vi "Cast Sensor Data.vi"(5 "SubPort":i32, 6 "Signal Type":enum16{"Digital", "Analog"}(ring), 7 "Port":i32, 8 "error IN":errorcluster, 9 "Key":string, 10 "Modbus Reading":u16[](array[numeric]), 11 "Data IN":map{string, dbl}(c390)) -> (0 "error OUT":errorcluster, 3 "Data OUT":map{string, dbl}(c390))   [LabVIEW 2024, in "IOLink.lvlib"]
uses:
  IOLink.lvlib
panel:
  out "Invalid":bool
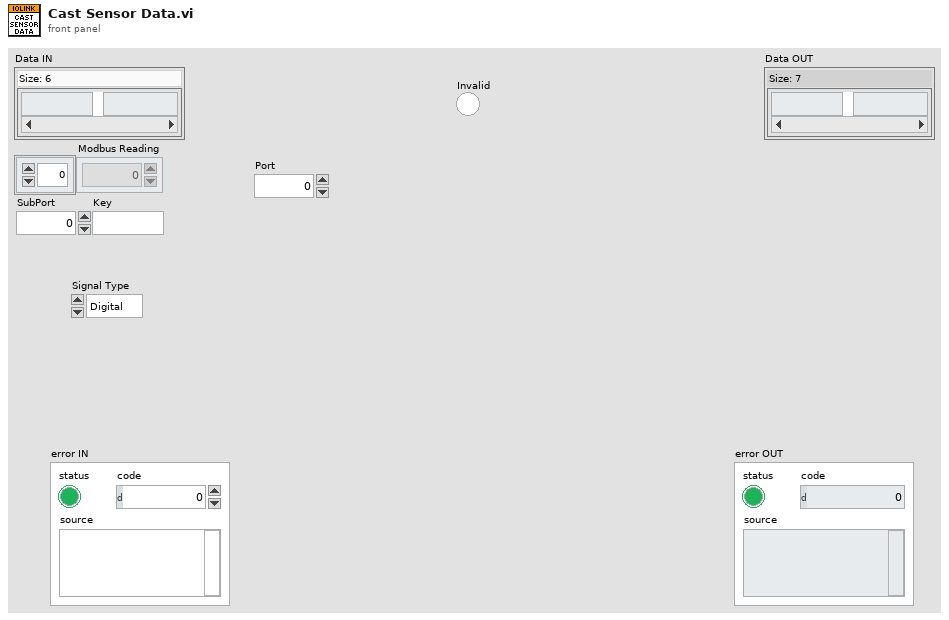
[diagram p1: front panel]
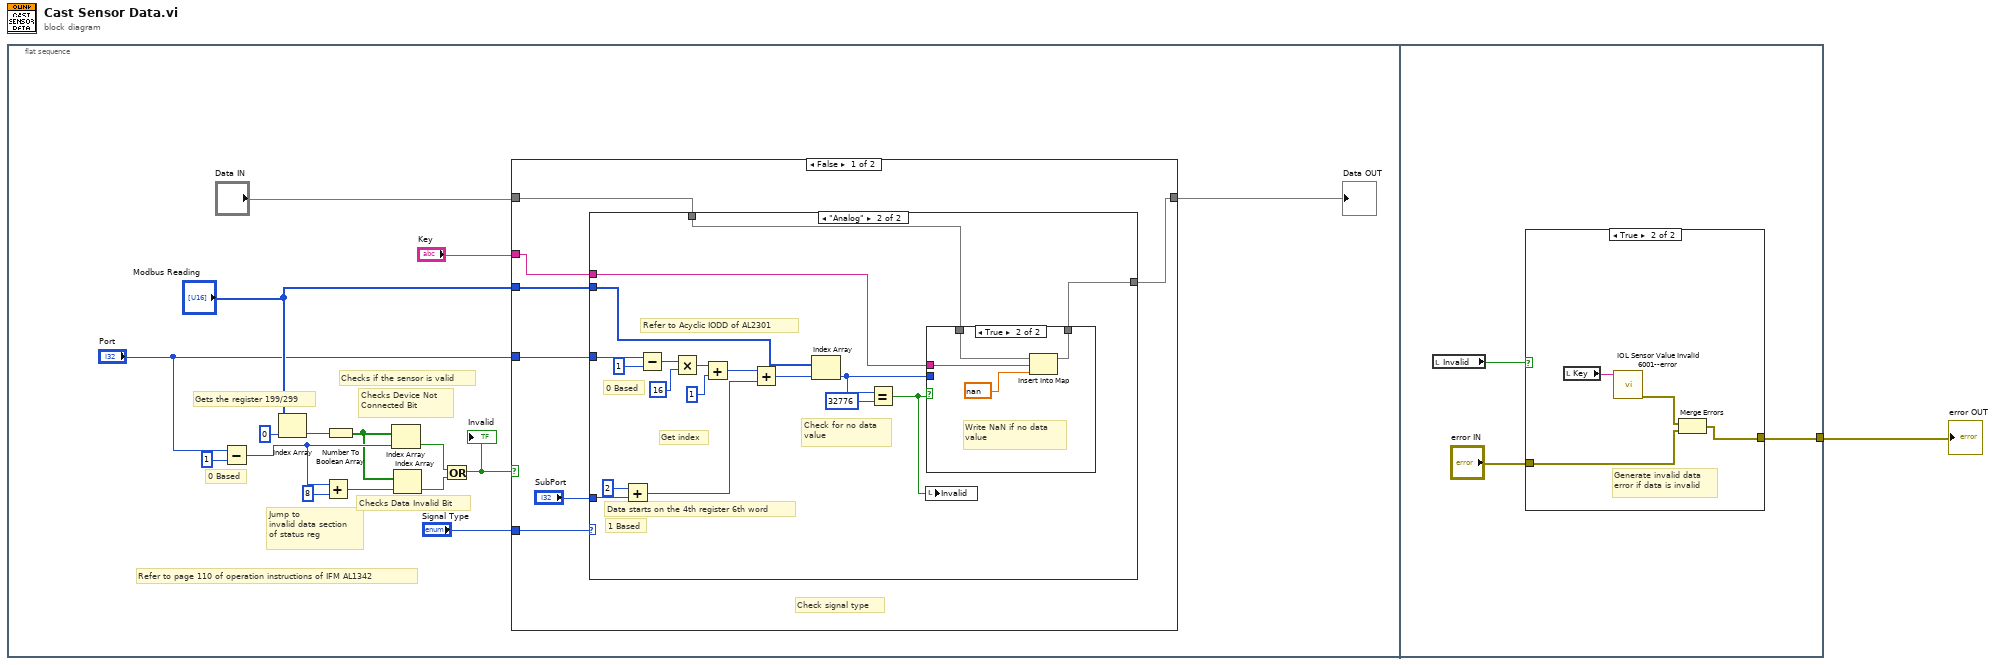
[diagram p0: block diagram]
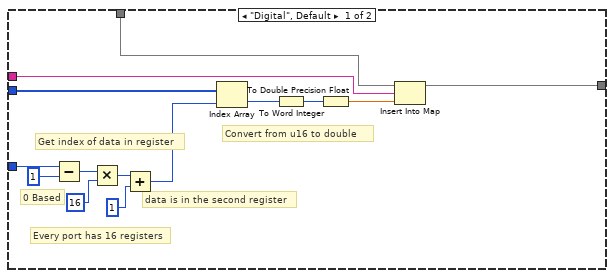
[diagram p2: hidden frame]
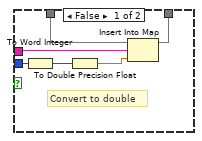
[diagram p3: hidden frame]
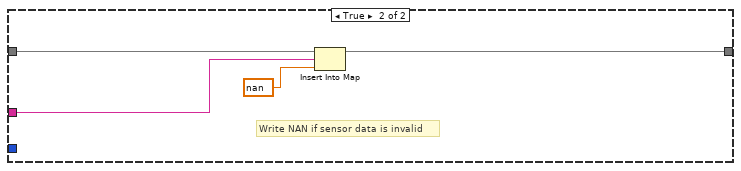
[diagram p4: hidden frame]
diagram:
  n1 = flat-sequence {
    tunnel: [w71] -> w1
    frame #0 {
      # "Checks Data Invalid Bit"
      # "Checks Device Not\nConnected Bit"
      # "Refer to page 110 of operation instructions of IFM AL1342"
      # "Jump to \ninvalid data section\nof status reg"
      # "0 Based"
      # "Gets the register 199/299"
      # "Checks if the sensor is valid"
      n2 = Subtract(x="Port", y=1) -> (x-y=w14:i32)
      n3 = Index Array(array="Modbus Reading", index=0) -> (element=w12:u16)
      n4 = Add(x=w14, y=8) -> (x+y=w15:i32)
      n5 = Number To Boolean Array(number=w12) -> (Boolean array=w13:bool[])
      n6 = Index Array(array=w13, index=w14) -> (element=w16:bool)
      n7 = Index Array(array=w13, index=w15) -> (element=w17:bool)
      n8 = Or(x=w16, y=w17) -> (x .or. y?=w5:bool)
      "Invalid" <- w5
      n9 = case shown="False" w5 {
        tunnel: "Signal Type" -> [w24 _]
        tunnel: "Modbus Reading" -> [w22 _]
        tunnel: "Port" -> [w21 _]
        tunnel: "Key" -> [w19 w69]
        tunnel: "Data IN" -> [w20 w70]
        tunnel: [w18 w67] -> w6
        frame False {
          # "Check signal type"
          n10 = case shown="\"Analog\"" w24 {
            tunnel: "SubPort" -> [_ w50]
            tunnel: w22 -> [w32 w45]
            tunnel: w21 -> [w38 w51]
            tunnel: w20 -> [w27 w43]
            tunnel: w19 -> [w26 w41]
            tunnel: [w25 w42] -> w18
            frame "Digital", Default {
              # "data is in the second register"
              # "Every port has 16 registers"
              # "0 Based"
              # "Convert from u16 to double"
              # "Get index of data in register"
              n11 = Subtract(x=w38, y=1) -> (x-y=w36:i32)
              n12 = Multiply(x=w36, y=16) -> (x*y=w34:i32)
              n13 = Add(x=w34, y=1) -> (x+y=w31:i32)
              n14 = Index Array(array=w32, index=w31) -> (element=w30:u16)
              n15 = To Word Integer(number=w30) -> (16bit integer=w29:i16)
              n16 = To Double Precision Float(number=w29) -> (double precision float=w28:dbl)
              n17 = Insert Into Map(map in=w27, key=w26, value=w28) -> (map out=w25:map{string, dbl})  [unwired: 2 out]
            }
            frame "Analog" {
              # "Refer to Acyclic IODD of AL2301"
              # "Data starts on the 4th register 6th word"
              # "1 Based"
              # "0 Based"
              # "Check for no data\nvalue"
              # "Get index"
              n18 = Add(x=2, y=w50) -> (x+y=w47:i32)
              n19 = Subtract(x=w51, y=1) -> (x-y=w55:i32)
              n20 = Multiply(x=w55, y=16) -> (x*y=w53:i32)
              n21 = Add(x=w53, y=1) -> (x+y=w48:i32)
              n22 = Add(x=w48, y=w47) -> (x+y=w46:i32)
              n23 = Index Array(array=w45, index=w46) -> (element=w40:u16)
              n24 = Equal?(x=w40, y=u16 32776) -> (x = y?=w39:bool)
              n25 = local write "Invalid"(w39) -> ()
              n26 = case shown="True" w39 {
                tunnel: w43 -> [w59 w65]
                tunnel: [w57 w64] -> w42
                tunnel: w41 -> [w60 w63]
                tunnel: w40 -> [w61 _]
                frame False {
                  # "Convert to double"
                  n27 = To Word Integer(number=w61) -> (16bit integer=w62:i16)
                  n28 = To Double Precision Float(number=w62) -> (double precision float=w58:dbl)
                  n29 = Insert Into Map(map in=w59, key=w60, value=w58) -> (map out=w57:map{string, dbl})  [unwired: 2 out]
                }
                frame True {
                  # "Write NaN if no data\nvalue"
                  n30 = Insert Into Map(map in=w65, key=w63, value=nan) -> (map out=w64:map{string, dbl})  [unwired: 2 out]
                }
              }
            }
          }
        }
        frame True {
          # "Write NAN if sensor data is invalid"
          n31 = Insert Into Map(map in=w70, key=w69, value=nan) -> (map out=w67:map{string, dbl})  [unwired: 2 out]
        }
      }
      "Data OUT" <- w6
    }
    frame #1 {
      n32 = local read "Invalid"() -> (w73:bool)
      n33 = case shown="True" w73 {
        tunnel: "error IN" -> [w74 w76]
        tunnel: [w74 w75] -> w71
        frame False {
        }
        frame True {
          # "Generate invalid data\nerror if data is invalid"
          n34 = local read "Key"() -> (w78:string)
          n35 = call "IOL Sensor Value Invalid 6001--error.vi"("Sensor Key"=w78) -> ("error out"=w77:errorcluster)  [unwired: 10 in]
          n36 = Merge Errors(w77, w76) -> (w75:errorcluster)
        }
      }
    }
  }
  "error OUT" <- w1
